vi "semafor_for_for.vi"() -> ()   [LabVIEW 2016]
panel:
  in  "Repetari":i32
  in  "Verde":i32
  in  "Galben":i32
  in  "Rosu":i32
  out "Verde":bool
  out "Galben":bool
  out "Rosu":bool
  out "Secunda":i32
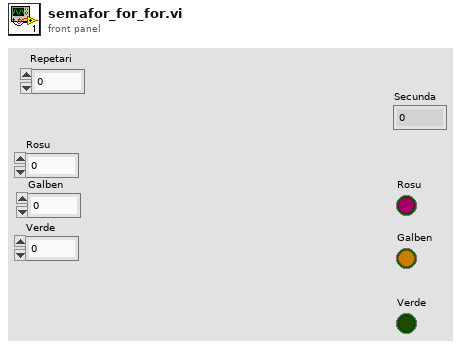
[diagram p1: front panel]
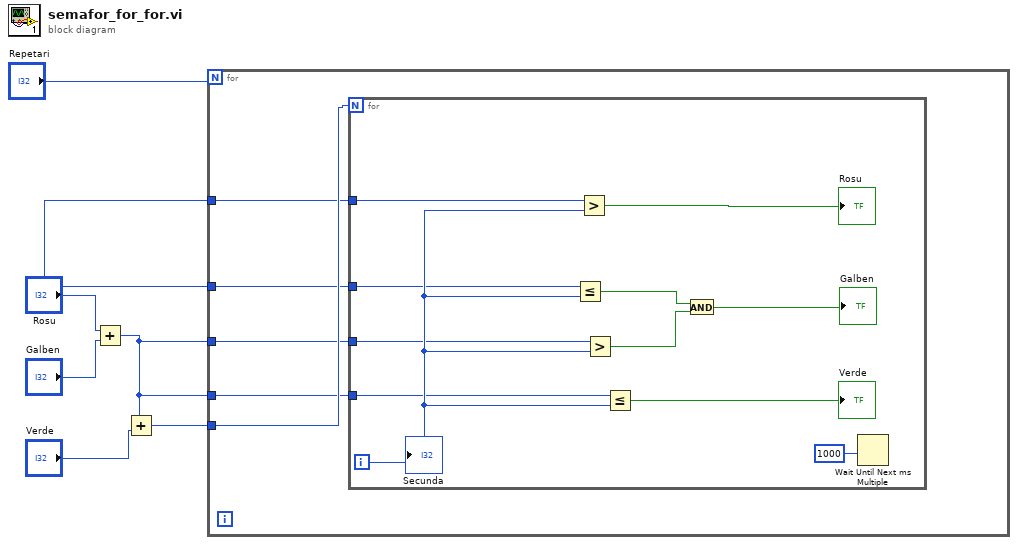
[diagram p0: block diagram]
diagram:
  n1 = Add(x="Rosu", y="Galben") -> (x+y=w2:i32)
  n2 = Add(x=w2, y="Verde") -> (x+y=w4:i32)
  n3 = for {
    N: "Repetari" -> [_]
    tunnel: w4 -> [w11]
    tunnel: "Rosu" -> [w10]
    tunnel: w2 -> [w9]
    tunnel: w2 -> [w8]
    tunnel: "Rosu" -> [w7]
    n4 = for {
      N: w11 -> [_]
      tunnel: w10 -> [w15]
      tunnel: w9 -> [w14]
      tunnel: w8 -> [w13]
      tunnel: w7 -> [w12]
      i -> [w17]
      n5 = Less Or Equal?(x=w12, y=w17) -> (x <= y?=w20:bool)
      n6 = Greater?(x=w15, y=w17) -> (0:→"Rosu":bool)
      n7 = Greater?(x=w13, y=w17) -> (0:w19:bool)
      n8 = Less Or Equal?(x=w14, y=w17) -> (x <= y?=→"Verde":bool)
      n9 = And(x=w20, y=w19) -> (x .and. y?=→"Galben":bool)
      n10 = Wait Until Next ms Multiple(millisecond multiple=u32 1000) -> ()  [unwired: 1 out]
      "Secunda" <- w17
    }
  }
